vi "量程参数写入.vi"(7 "error in (no error)":errorcluster caption="错误输入（无错误）", 9 "量程参数写入":T1, 10 "测量参数":u16(ring) items=["COD"=22, "氨氮"=3, "总氮"=2, "总磷"=1]) -> (0 "error out":errorcluster caption="错误输出")   [LabVIEW 2016, in "斯坦道氟化物.lvlib"]
uses:
  <vilib>/Plasmionique/MB Master/MB Master.lvlib
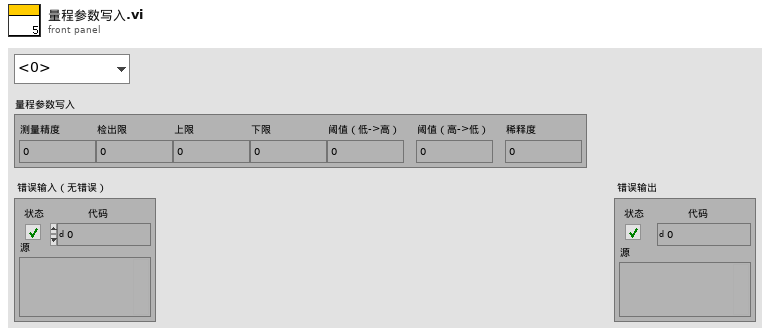
[diagram p1: front panel]
types:
  T1 = cluster{"测量精度":u16, "检出限":dbl, "上限":dbl, "下限":dbl, "阈值（低->高）":dbl, "阈值（高->低）":dbl, "稀释度":dbl}
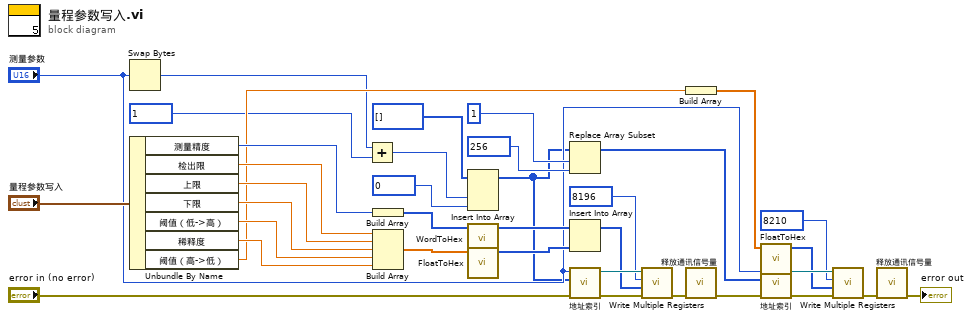
[diagram p0: block diagram]
diagram:
  n1 = Swap Bytes(anything="测量参数") -> (byte swapped=w17:u16)
  n2 = Unbundle By Name("量程参数写入") -> ("测量精度"=w32:u16, "检出限"=w31:dbl, "上限"=w30:dbl, "下限"=w29:dbl, "阈值（低->高）"=w28:dbl, "稀释度"=w27:dbl, "阈值（高->低）"=w23:dbl)
  n3 = Add(x=w17, y=u16 1 ("starting address")) -> (x+y=w21:u16)
  n4 = Build Array(w32) -> (w33:u16[])
  n5 = Build Array(w31, w30, w29, w28, w27) -> (w26:dbl[])
  n6 = Insert Into Array(array=u16[] [] ("数组"), new element #1=w21, new element #2=u16 0 ("starting address")) -> (w7:u16[])  [unwired: 1 in]
  n7 = call "WordToHex.vi"("WORD"=w33) -> ("数组"=w25:u16[])  [unwired: 10 in]
  n8 = call "FloatToHex.vi"("浮点数"=w26) -> ("DCBA整形输出"=w24:u16[])  [unwired: 10 in]
  n9 = Replace Array Subset(array=w7, new element=u16 256 ("starting address"), index=1 ("索引")) -> (w4:u16[])
  n10 = Insert Into Array(array=w25, new element=w24) -> (w5:u16[])  [unwired: 1 in]
  n11 = call "地址索引.vi"("error in (no error)"="error in (no error)", "values"=w7, "测量参数"="测量参数") -> ("error out"=w15:errorcluster, "MB session out"=w14:refnum<class "MB_Master.lvclass">)  [unwired: 7 in]
  n12 = call <vilib>:"Write Multiple Registers.vi"("error in (no error)"=w15, "values"=w5, "starting address"=u16 8196, "MB session in"=w14) -> ("error out"=w13:errorcluster)  [unwired: 6 in, 1 out]
  n13 = Build Array(w23) -> (w22:dbl[])
  n14 = call "释放通讯信号量.vi"("error in (no error)"=w13) -> ("error out"=w9:errorcluster)  [unwired: 10 in]
  n15 = call "FloatToHex.vi"("浮点数"=w22) -> ("DCBA整形输出"=w2:u16[])  [unwired: 10 in]
  n16 = call "地址索引.vi"("error in (no error)"=w9, "values"=w4, "测量参数"="测量参数") -> ("error out"=w10:errorcluster, "MB session out"=w11:refnum<class "MB_Master.lvclass">)  [unwired: 7 in]
  n17 = call <vilib>:"Write Multiple Registers.vi"("error in (no error)"=w10, "values"=w2, "starting address"=u16 8210, "MB session in"=w11) -> ("error out"=w12:errorcluster)  [unwired: 6 in, 1 out]
  n18 = call "释放通讯信号量.vi"("error in (no error)"=w12) -> ("error out"=→"error out":errorcluster)  [unwired: 10 in]
